vi "AddCurveArrDev.vi"(6 "ArrDevDat":T1[](array[typedef]), 8 "error in":errorcluster caption="entrée d'erreur (pas d'erreur)", 9 "CurPointInd":i32, 10 "Exper.lvclass In":refnum<class "Experiment.lvclass">, 11 "InterfaceIn":refnum<class "Interface.lvclass">) -> (0 "error out":errorcluster caption="sortie d'erreur", 3 "InterfaceOut":refnum<class "Interface.lvclass">)   [LabVIEW 2019, in "Interface.lvclass"]
uses:
  Interface.lvclass
  Experiment Class/Experiment.lvclass
  Experiment Class/ArrDevData.ctl
  CurveSetup.ctl
  AddCurveStatesArrDev.ctl
  ScanParams.ctl
  Interface.lvclass/Interface.ctl
panel:
  out "ReuseVarPar":bool
  out "DataFileName":path
  out "IndInGraphCrv":i32[](array[numeric])
  out "CurrDataQ":refnum<queue>[](array[refnum])
  out "CurrVarParQ":refnum<queue>[](array[refnum])
  out "Scan list":string[](array[string])
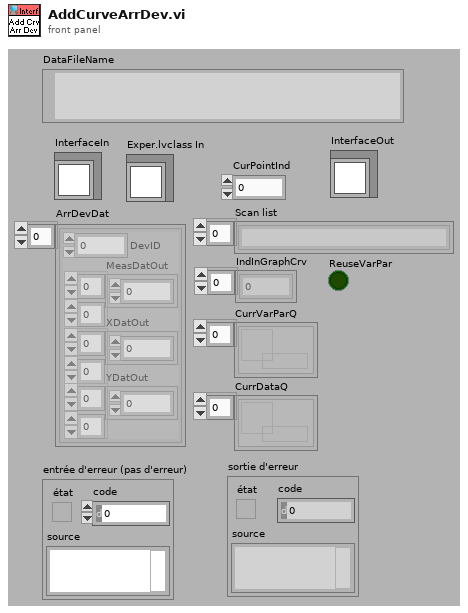
[diagram p1: front panel]
types:
  T1 = typedef "ArrDevData.ctl" = cluster{"MeasDatOut":dbl[][], "XDatOut":dbl[][], "YDatOut":dbl[][], "DevID":i32}
  T2 = typedef "Interface.lvclass/CurveSetup.ctl" = cluster{"CurveName":string, "YParam":string, "XParam":string, "ZParam ":string, "GroupName":string, "LinWdth":u8, "PntCol":u32, "LinCol":u32, "LablFor":u8, "XScale":u32, "YScale":u32, "Interpol":u8, "DisplayName":string, "FillType":i16, "LineStyle":u8, "PntStyle":u8, "BarTyp":u8, "GraphIndex":i32, "Visible":bool, "XScaleName":string, "YScaleName":string, "XYGraph_Ref":refnum<vi>, "Data Only":bool, "DataQ Ref":refnum<queue>, "XParQ Ref":refnum<queue>, "XParamInd":i32, "ScanInd":i32}
  T3 = typedef "Interface.lvclass/ScanParams.ctl" = cluster{"Entête":string, "Scan list":string[], "NbCourbe":i32, "IndCourbe":i64, "NomDon":string[], "Session ":i32, "Date":string, "Time":string, "VarParams":string[][], "UserName":string, "ScanTableSize":i32[], "VarPar list":string[], "DescKeyword":string}
  T4 = typedef "AddCurveStatesArrDev.ctl" = enum16{"CreateCurvePar", "AddToGraph", "AddToCrvParArr", "CreateDataQ", "UpdateGraph", "Error"}
  T5 = enum16{"open", "replace", "create", "open or create", "replace or create", "replace or create with confirmation"}
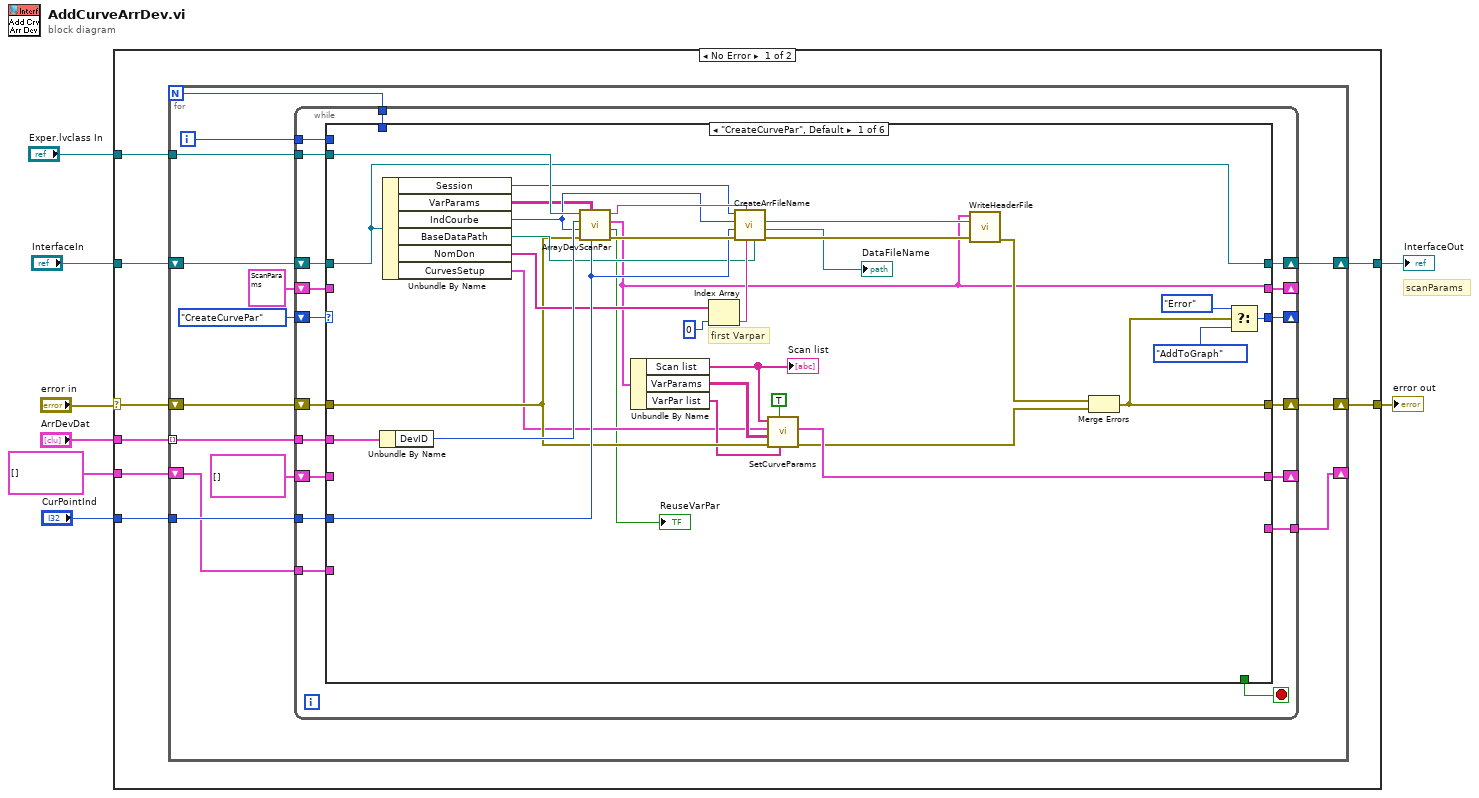
[diagram p0: block diagram]
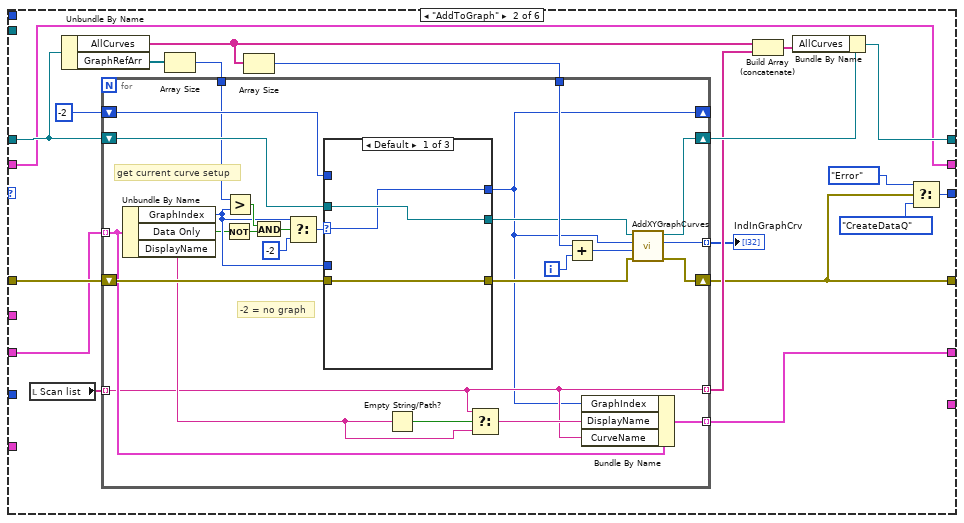
[diagram p2: hidden frame]
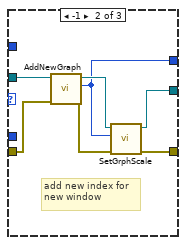
[diagram p3: hidden frame]
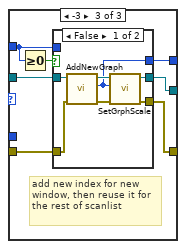
[diagram p4: hidden frame]
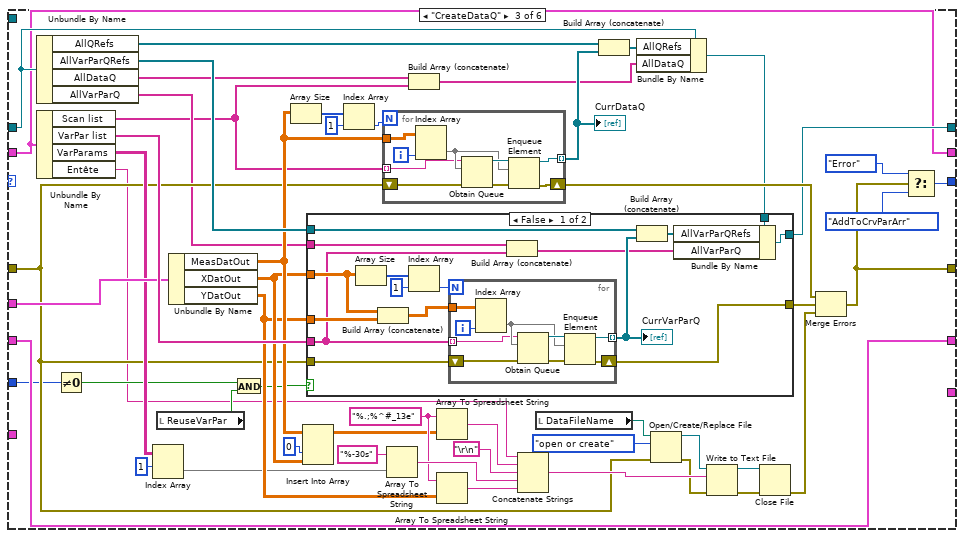
[diagram p6: hidden frame]
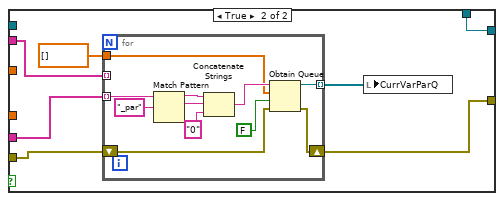
[diagram p7: hidden frame]
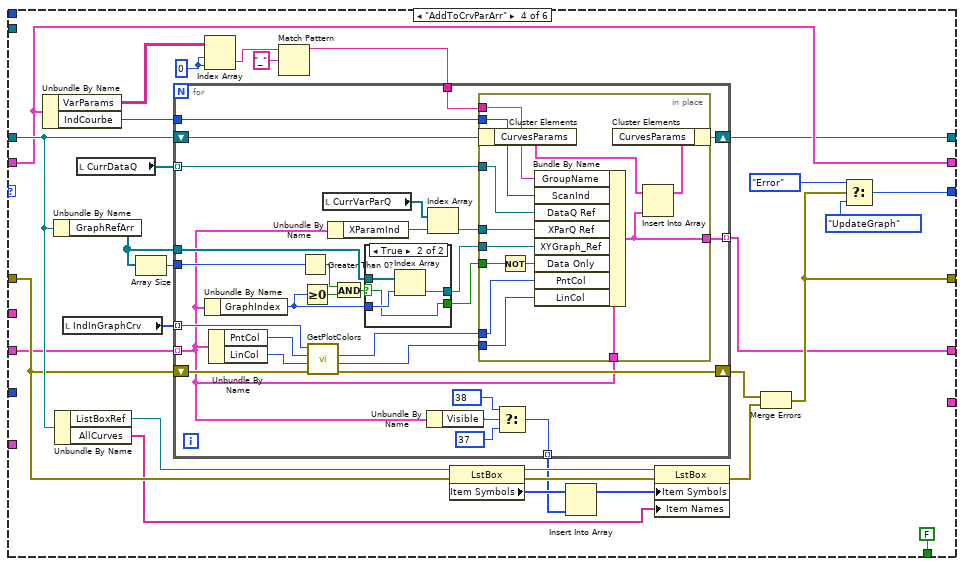
[diagram p8: hidden frame]
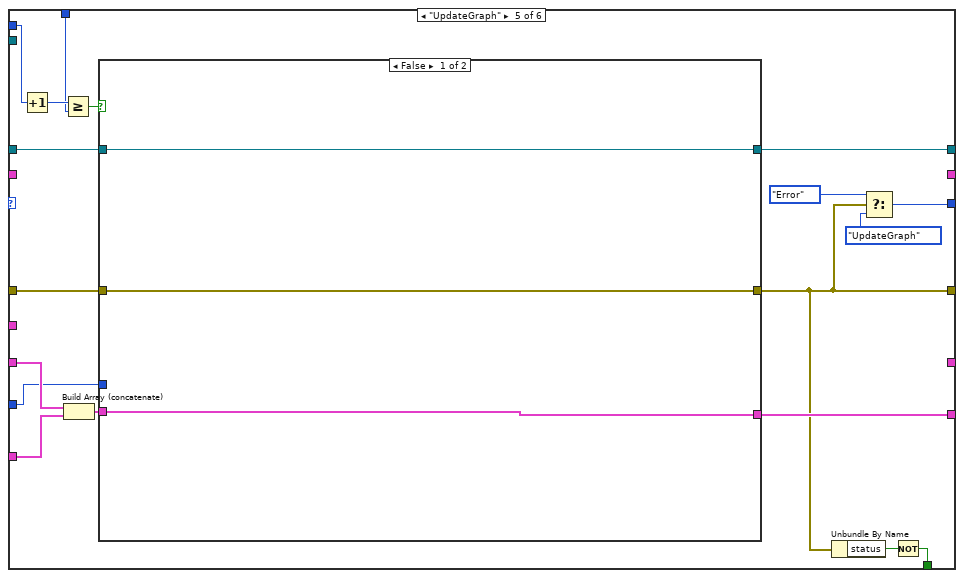
[diagram p10: hidden frame]
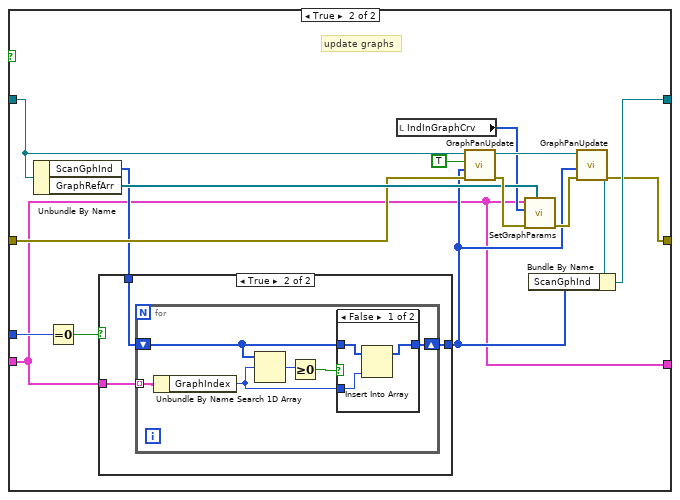
[diagram p11: hidden frame]
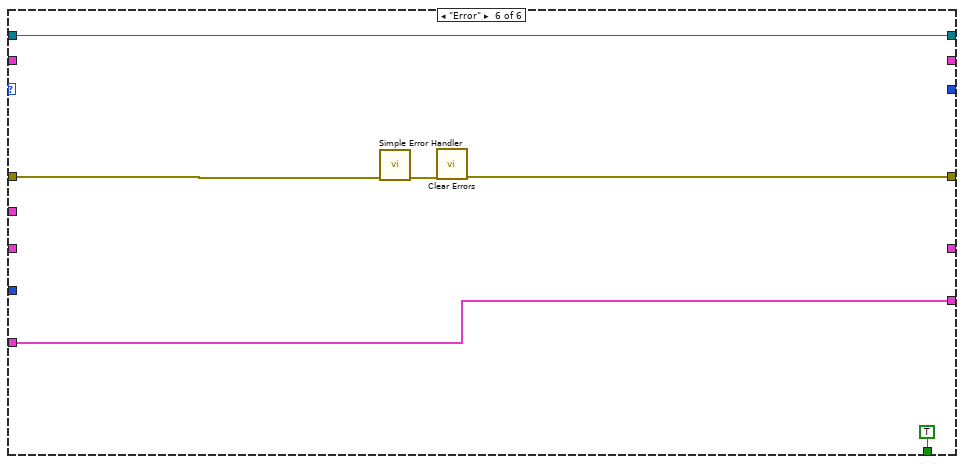
[diagram p14: hidden frame]
diagram:
  # "scanParams"
  n1 = case shown="No Error" "error in" {
    selector: "error in" -> [w16 w393]
    tunnel: [w15 w393] -> w7
    tunnel: "InterfaceIn" -> [w13 w392]
    tunnel: [w14 w392] -> w5
    tunnel: "ArrDevDat" -> [w12 _]
    tunnel: "Exper.lvclass In" -> [w11 _]
    tunnel: "CurPointInd" -> [w10 _]
    tunnel: T2[] [] ("CurveSetupsOut") -> [w9 _]
    frame No Error {
      n2 = for {
        N -> [w18]
        tunnel: w12 -> [w26] mode=indexing
        tunnel: w11 -> [w24]
        tunnel: w10 -> [w23]
        shift-right: [w29] -> w15
        shift-left: w16 -> [w30]
        shift-right: [w28] -> w14
        shift-left: w13 -> [w27]
        shift-right: [w19] -> _
        shift-left: w9 -> [w20]
        i -> [w17]
        n3 = while {
          shift-right: [w44] -> w29
          shift-left: w30 -> [w46]
          shift-right: [w45] -> _
          shift-left: AddCurveStatesArrDev."CreateCurvePar" ("Énum") -> [w47]
          shift-right: [w43] -> w28
          shift-left: w27 -> [w42]
          shift-right: [w41] -> _
          shift-left: T2[] [] ("CurveSetupsOut") -> [w40]
          tunnel: w26 -> [w39]
          tunnel: w24 -> [w38]
          tunnel: w23 -> [w37]
          shift-right: [w36] -> _
          shift-left: T3 {"Entête"="", "Scan list"=[], "NbCourbe"=1, "IndCourbe"=0, "NomDon"=["RTêta;", "X&Y;"], "Session "=0, "Date"="", "Time"="", "VarParams"=[], "UserName"="", "ScanTableSize"=[], "VarPar list"=[], "DescKeyword"=""} ("ScanPar") -> [w35]
          tunnel: w20 -> [w34]
          tunnel: [w33] -> w19
          tunnel: w18 -> [w32]
          tunnel: w17 -> [w31]
          stop <- w48 stop-if-true
          n4 = case shown="\"CreateCurvePar\", Default" w47 {
            tunnel: [_ _ _ FALSE w338 TRUE] -> w48
            tunnel: w46 -> [w64 w100 w168 w273 w352 w389]
            tunnel: w42 -> [w50 w96 w192 w285 w350 w387]
            tunnel: [w52 w84 w166 w264 w339 _] -> w45
            tunnel: [w54 w82 w164 w261 w337 w388] -> w44
            tunnel: [w50 w98 w194 w260 w351 w387] -> w43
            tunnel: [w60 w87 w169 w259 _ _] -> w41
            tunnel: w40 -> [_ w94 w169 w267 w349 _]
            tunnel: w39 -> [w79 _ w198 _ _ _]
            tunnel: w38 -> [w80 _ _ _ _ _]
            tunnel: w37 -> [w73 _ w162 _ w335 _]
            tunnel: [w63 w81 w163 w268 _ _] -> w36
            tunnel: w35 -> [_ w81 w163 w268 _ _]
            tunnel: w34 -> [_ _ _ _ w348 w386]
            tunnel: [_ _ _ _ w347 w386] -> w33
            tunnel: w32 -> [_ _ _ _ w344 _]
            tunnel: w31 -> [_ _ _ _ w343 _]
            frame "CreateCurvePar", Default {
              # "first Varpar"
              n5 = Unbundle By Name(w79) -> ("DevID"=w78:i32)
              n6 = Unbundle By Name(w50) -> ("Session"=w69:i32, "VarParams"=w66:string[][], "IndCourbe"=w72:i64, "BaseDataPath"=w68:path, "NomDon"=w65:string[], "CurvesSetup"=w57:T2[])
              n7 = call "ArrayDevScanPar.vi"("CurPointInd"=w73, "VarParams"=w66, "error in"=w64, "IndCourbe"=w72, "DevID"=w78, "Experiment.lvclass In"=w80) -> ("error out"=w77:errorcluster, "ReuseVarPar"=→"ReuseVarPar":bool, "ScanPar"=w63:T3, "FileNmDTString"=w76:string)  [unwired: 2 in]
              n8 = Unbundle By Name(w63) -> ("Scan list"=w58:string[], "VarParams"=w62:string[][], "VarPar list"=w61:string[])
              "Scan list" <- w58
              n9 = Index Array(array=w65, index=0 ("indice (ligne)")) -> (element=w74:string)
              n10 = call "CreateArrFileName.vi"("BaseDataPath"=w68, "VarParName"=w74, "Date"=w76, "error in (no error)"=w77, "PointIndex"=w73, "ScanIndex"=w72, "SessionInd"=w69) -> ("error out"=w71:errorcluster, "DataFileName"=→"DataFileName":path, "HeadersFileName"=w70:path)  [unwired: 2 in]
              n11 = call "SetCurveParams.vi"("VarPar list"=w61, "AllowDef"=TRUE, "error in (no error)"=w64, "VarParams"=w62, "CurveSetupsIn"=w57, "CurveNames"=w58) -> ("error out"=w59:errorcluster, "CurveSetupsOut"=w60:T2[])  [unwired: 4 in]
              n12 = call "WriteHeaderFile.vi"("error in (no error)"=w71, "HeadersFileName"=w70, "ScanPar"=w63) -> ("error out"=w67:errorcluster)  [unwired: 8 in]
              n13 = Merge Errors(w67, w59) -> (w54:errorcluster)
              n14 = Select(t=AddCurveStatesArrDev."Error" ("Énum"), s=w54, f=AddCurveStatesArrDev."AddToGraph" ("Énum")) -> (s? t:f=w52:T4)
            }
            frame "AddToGraph" {
              n15 = local read "Scan list"() -> (w88:string[])
              n16 = Unbundle By Name(w96) -> ("AllCurves"=w91:string[], "GraphRefArr"=w93:refnum<vi>[])
              n17 = Array Size(array=w93) -> (size(s)=w92:i32)
              n18 = Array Size(array=w91) -> (size(s)=w95:i32)
              n19 = for {
                tunnel: w94 -> [w118] mode=indexing
                shift-right: [w102] -> _
                shift-left: -2 ("NewGraphInd") -> [w117]
                shift-right: [w106] -> w99
                shift-left: w96 -> [w116]
                tunnel: w95 -> [w108]
                tunnel: w92 -> [w115]
                tunnel: [w110] -> w89 mode=indexing
                tunnel: [w114] -> w87 mode=indexing
                tunnel: w88 -> [w110] mode=indexing
                shift-right: [w104] -> w82
                shift-left: w100 -> [w119]
                tunnel: [w101] -> w86 mode=indexing
                i -> [w109]
                # "-2 = no graph"
                # "get current curve setup"
                n20 = Unbundle By Name(w118) -> ("GraphIndex"=w125:i32, "Data Only"=w122:bool, "DisplayName"=w112:string)
                n21 = Not(x=w122) -> (.not. x?=w121:bool)
                n22 = Greater?(x=w115, y=w125) -> (0:w126:bool)
                n23 = And(x=w126, y=w121) -> (x .and. y?=w120:bool)
                n24 = Select(t=w125, s=w120, f=-2 ("cas faux")) -> (s? t:f=w123:i32)
                n25 = case shown="Default" w123 {
                  selector: w123 -> [w127 _ _]
                  tunnel: w125 -> [_ _ _]
                  tunnel: [w127 w130 w139] -> w102
                  tunnel: w116 -> [w129 w136 w143]
                  tunnel: w119 -> [w128 w135 w142]
                  tunnel: [w129 w133 w141] -> w107
                  tunnel: [w128 w131 w140] -> w105
                  tunnel: w117 -> [_ _ w137]
                  frame Default {
                  }
                  frame -1 {
                    # "add new index for new window"
                    n26 = call "AddNewGraph.vi"("error in (no error)"=w135, "Interface en entrée"=w136) -> ("error out"=w132:errorcluster, "NewGraphInd"=w130:i32, "Interface en sortie"=w134:refnum<class "Interface.lvclass">)  [unwired: 7 in]
                    n27 = call "SetGrphScale.vi"("error in (no error)"=w132, "GraphIndex"=w130, "Interface en entrée"=w134) -> ("error out"=w131:errorcluster, "Interface en sortie"=w133:refnum<class "Interface.lvclass">)  [unwired: 7 in]
                  }
                  frame -3 {
                    # "add new index for new window, then reuse it for the rest of scanlist"
                    n28 = Greater Or Equal To 0?(x=w137) -> (x >= 0?=w138:bool)
                    n29 = case shown="False" w138 {
                      tunnel: w143 -> [w150 w153]
                      tunnel: w142 -> [w149 w152]
                      tunnel: [w147 w153] -> w141
                      tunnel: [w145 w152] -> w140
                      tunnel: [w144 w151] -> w139
                      tunnel: w137 -> [_ w151]
                      frame False {
                        n30 = call "AddNewGraph.vi"("error in (no error)"=w149, "Interface en entrée"=w150) -> ("error out"=w146:errorcluster, "NewGraphInd"=w144:i32, "Interface en sortie"=w148:refnum<class "Interface.lvclass">)  [unwired: 7 in]
                        n31 = call "SetGrphScale.vi"("error in (no error)"=w146, "GraphIndex"=w144, "Interface en entrée"=w148) -> ("error out"=w145:errorcluster, "Interface en sortie"=w147:refnum<class "Interface.lvclass">)  [unwired: 7 in]
                      }
                      frame True {
                      }
                    }
                  }
                }
                n32 = Empty String/Path?(string/path=w112) -> (empty?=w113:bool)
                n33 = Select(t=w110, s=w113, f=w112) -> (s? t:f=w111:string)
                n34 = Add(x=w108, y=w109) -> (x+y=w103:i32)
                n35 = Bundle By Name(cluster=w118, "GraphIndex"=w102, "DisplayName"=w111, "CurveName"=w110) -> (w114:T2)
                n36 = call "AddXYGraphCurves.vi"("error in (no error)"=w105, "CurvIndex"=w103, "GraphIndex"=w102, "Interface en entrée"=w107) -> ("error out"=w104:errorcluster, "IndInGrphCrv"=w101:i32, "Interface en sortie"=w106:refnum<class "Interface.lvclass">)  [unwired: 5 in]
              }
              "IndInGraphCrv" <- w86
              n37 = Build Array (concatenate)(w91, w89) -> (w90:string[])
              n38 = Bundle By Name(cluster=w99, "AllCurves"=w90) -> (w98:refnum<class "Interface.lvclass">)
              n39 = Select(t=AddCurveStatesArrDev."Error" ("Énum"), s=w82, f=AddCurveStatesArrDev."CreateDataQ" ("Énum")) -> (s? t:f=w84:T4)
            }
            frame "CreateDataQ" {
              w185 = "%.;%^#_13e" ("chaîne de format")
              n40 = Unbundle By Name(w192) -> ("AllQRefs"=w193:refnum<queue>[], "AllVarParQRefs"=w200:refnum<queue>[], "AllDataQ"=w156:string[], "AllVarParQ"=w158:string[])
              n41 = Unbundle By Name(w163) -> ("Scan list"=w155:string[], "VarPar list"=w199:string[], "VarParams"=w177:string[][], "Entête"=w157:string)
              n42 = Not Equal To 0?(x=w162) -> (x != 0?=w159:bool)
              n43 = Index Array(array=w177, index (row)=1 ("indice (ligne)")) -> (element=w175:string[])  [unwired: 1 in]
              n44 = local read "ReuseVarPar"() -> (w160:bool)
              n45 = Unbundle By Name(w198) -> ("MeasDatOut"=w190:dbl[][], "XDatOut"=w180:dbl[][], "YDatOut"=w178:dbl[][])
              n46 = And(x=w159, y=w160) -> (x .and. y?=w161:bool)
              n47 = Array Size(array=w190) -> (size(s)=w205:i32[])
              n48 = Insert Into Array(array=w190, index (col)=0 ("indice désactivé (col)"), new element=w180) -> (w179:dbl[][])  [unwired: 1 in]
              n49 = Index Array(array=w205, index=1 ("indice")) -> (element=w203:i32)
              n50 = for {
                N: w203 -> [_]
                tunnel: w190 -> [w256]
                shift-right: [w257] -> w196
                shift-left: w168 -> [w251]
                tunnel: [w252] -> w202 mode=indexing
                tunnel: w155 -> [w250] mode=indexing
                i -> [w249]
                n51 = Index Array(array=w256, index (col)=w249) -> (element=w253:dbl[])  [unwired: 1 in]
                n52 = Obtain Queue(name (unnamed)=w250, element data type=w253, error in (no error)=w251) -> (queue out=w255:refnum<queue>, error out=w254:errorcluster)  [unwired: 2 in, 1 out]
                n53 = Enqueue Element(queue=w255, element=w253, error in (no error)=w254) -> (queue out=w252:refnum<queue>, error out=w257:errorcluster)  [unwired: 1 in, 1 out]
              }
              "CurrDataQ" <- w202
              n54 = Array To Spreadsheet String(array=w175, 3:"%-30s" ("chaîne de format")) -> (spreadsheet string=w188:string)  [unwired: 1 in]
              n55 = Build Array (concatenate)(w156, w155) -> (w154:string[])
              n56 = Array To Spreadsheet String(array=w179, 3:w185) -> (spreadsheet string=w186:string)  [unwired: 1 in]
              n57 = Array To Spreadsheet String(array=w178, 3:w185) -> (spreadsheet string=w181:string)  [unwired: 1 in]
              n58 = Concatenate Strings(w157, w186, "\r\n", w188, w181) -> (w182:string)
              n59 = local read "DataFileName"() -> (w171:path)
              n60 = Build Array (concatenate)(w193, w202) -> (w201:refnum<queue>[])
              n61 = Bundle By Name(cluster=w192, "AllQRefs"=w201, "AllDataQ"=w154) -> (w195:refnum<class "Interface.lvclass">)
              n62 = case shown="False" w161 {
                tunnel: w180 -> [w211 _]
                tunnel: w200 -> [w210 _]
                tunnel: w178 -> [w216 _]
                tunnel: w199 -> [w208 w236]
                tunnel: w168 -> [w215 w234]
                tunnel: [w209 w231] -> w197
                tunnel: w195 -> [w214 w237]
                tunnel: [w213 w237] -> w194
                tunnel: w158 -> [w207 w235]
                frame False {
                  n63 = Array Size(array=w211) -> (size(s)=w219:i32[])
                  n64 = Build Array (concatenate)(w211, w216) -> (w217:dbl[][])
                  n65 = Index Array(array=w219, index=1 ("indice")) -> (element=w221:i32)
                  n66 = for {
                    N: w221 -> [_]
                    tunnel: w217 -> [w229]
                    shift-right: [w230] -> w209
                    shift-left: w215 -> [w224]
                    tunnel: [w225] -> w218 mode=indexing
                    tunnel: w208 -> [w223] mode=indexing
                    i -> [w222]
                    n67 = Index Array(array=w229, index (col)=w222) -> (element=w226:dbl[])  [unwired: 1 in]
                    n68 = Obtain Queue(name (unnamed)=w223, element data type=w226, error in (no error)=w224) -> (queue out=w228:refnum<queue>, error out=w227:errorcluster)  [unwired: 2 in, 1 out]
                    n69 = Enqueue Element(queue=w228, element=w226, error in (no error)=w227) -> (queue out=w225:refnum<queue>, error out=w230:errorcluster)  [unwired: 1 in, 1 out]
                  }
                  "CurrVarParQ" <- w218
                  n70 = Build Array (concatenate)(w207, w208) -> (w206:string[])
                  n71 = Build Array (concatenate)(w210, w218) -> (w212:refnum<queue>[])
                  n72 = Bundle By Name(cluster=w214, "AllVarParQRefs"=w212, "AllVarParQ"=w206) -> (w213:refnum<class "Interface.lvclass">)
                }
                frame True {
                  n73 = for {
                    tunnel: w236 -> [w247] mode=indexing
                    tunnel: w235 -> [_] mode=indexing
                    tunnel: [w242] -> w232 mode=indexing
                    shift-right: [w240] -> w231
                    shift-left: w234 -> [w241]
                    tunnel: dbl[] [] ("sous-tableau") -> [w239]
                    n74 = Match Pattern(string=w247, regular expression="_par" ("expression régulière")) -> (before substring=w246:string, match substring=w245:string)  [unwired: 1 in, 2 out]
                    n75 = Concatenate Strings(w246, w245, "0" ("chaîne")) -> (w243:string)
                    n76 = Obtain Queue(name (unnamed)=w243, element data type=w239, create if not found? (T)=FALSE ("créer si introuvable ? (V)"), error in (no error)=w241) -> (queue out=w242:refnum<queue>, error out=w240:errorcluster)  [unwired: 1 in, 1 out]
                  }
                  n77 = local write "CurrVarParQ"(w232) -> ()
                }
              }
              n78 = Open/Create/Replace File(file path (use dialog)=w171, error in=w168, operation (0:open)=T5."open or create" ("opération (0 : open)")) -> (refnum out=w170:refnum<file>, error out=w172:errorcluster)  [unwired: 3 in, 1 out]
              n79 = Write to Text File(file (use dialog)=w170, text=w182, error in=w172) -> (refnum out=w184:refnum<file>, error out=w183:errorcluster)  [unwired: 1 in, 1 out]
              n80 = Close File(refnum=w184, error in=w183) -> (error out=w174:errorcluster)  [unwired: 1 out]
              n81 = Merge Errors(w196, w197, w174) -> (w164:errorcluster)
              n82 = Select(t=AddCurveStatesArrDev."Error" ("Énum"), s=w164, f=AddCurveStatesArrDev."AddToCrvParArr" ("Énum")) -> (s? t:f=w166:T4)
            }
            frame "AddToCrvParArr" {
              w280 = 0 ("indice désactivé (col)")
              n83 = Unbundle By Name(w268) -> ("VarParams"=w281:string[][], "IndCourbe"=w282:i64)
              n84 = Unbundle By Name(w285) -> ("GraphRefArr"=w284:refnum<vi>[])
              n85 = Unbundle By Name(w285) -> ("ListBoxRef"=w276:refnum<vi>, "AllCurves"=w265:string[])
              n86 = local read "IndInGraphCrv"() -> (w287:i32[])
              n87 = local read "CurrDataQ"() -> (w283:refnum<queue>[])
              n88 = Array Size(array=w284) -> (size(s)=w286:i32)
              n89 = Index Array(array=w281, index (row)=w280, index (col)=w280) -> (element=w279:string)
              n90 = Match Pattern(string=w279, regular expression="_" ("expression régulière")) -> (before substring=w277:string)  [unwired: 1 in, 3 out]
              n91 = for {
                tunnel: w267 -> [w291] mode=indexing
                tunnel: w287 -> [w308] mode=indexing
                tunnel: w284 -> [w305]
                tunnel: w286 -> [w304]
                tunnel: w283 -> [w302] mode=indexing
                tunnel: w282 -> [w297]
                tunnel: w277 -> [w290]
                tunnel: [w293] -> w271 mode=indexing
                shift-right: [w292] -> w266
                shift-left: w273 -> [w313]
                shift-right: [w289] -> w260
                shift-left: w285 -> [w316]
                tunnel: [w288] -> w259 mode=indexing
                n92 = Unbundle By Name(w291) -> ("GraphIndex"=w312:i32)
                n93 = Unbundle By Name(w291) -> ("PntCol"=w314:u32, "LinCol"=w315:u32)
                n94 = Greater Than 0?(x=w304) -> (x > 0?=w309:bool)
                n95 = Greater Or Equal To 0?(x=w312) -> (x >= 0?=w310:bool)
                n96 = call "GetPlotColors.vi"("ErrorIn(No Error)"=w313, "Color2In"=w315, "Color1In"=w314, "ColorIndex"=w308) -> ("sortie d'erreur"=w292:errorcluster, "Color2Out"=w307:u32, "Color1Out"=w306:u32)  [unwired: 4 in, 1 out]
                n97 = local read "CurrVarParQ"() -> (w300:refnum<queue>[])
                n98 = Unbundle By Name(w291) -> ("XParamInd"=w301:i32)
                n99 = And(x=w309, y=w310) -> (x .and. y?=w311:bool)
                n100 = case shown="True" w311 {
                  selector: w311 -> [w317 w318]
                  tunnel: [_ w321] -> w298
                  tunnel: w305 -> [_ w320]
                  tunnel: w312 -> [_ w319]
                  tunnel: [w317 w318] -> w303
                  frame False {
                  }
                  frame True {
                    n101 = Index Array(array=w320, index=w319) -> (element=w321:refnum<vi>)
                  }
                }
                n102 = Unbundle By Name(w291) -> ("Visible"=w296:bool)
                n103 = Index Array(array=w300, index=w301) -> (element=w299:refnum<queue>)
                n104 = in-place {
                  in-place-border: w307 -> [w325]
                  in-place-border: w306 -> [w324]
                  in-place-border: w298 -> [w332]
                  in-place-border: w303 -> [w331]
                  in-place-border: w302 -> [w330]
                  in-place-border: w299 -> [w329]
                  in-place-border: w297 -> [w327]
                  in-place-border: w291 -> [w328]
                  in-place-border: w290 -> [w326]
                  in-place-border: [w322] -> w288
                  n105 = in-place-cluster #1(w316) -> ("CurvesParams"=w334:T2[])
                  n106 = Not(x=w331) -> (.not. x?=w323:bool)
                  n107 = Bundle By Name(cluster=w328, "GroupName"=w326, "ScanInd"=w327, "DataQ Ref"=w330, "XParQ Ref"=w329, "XYGraph_Ref"=w332, "Data Only"=w323, "PntCol"=w324, "LinCol"=w325) -> (w322:T2)
                  n108 = Insert Into Array(array=w334, new element=w322) -> (w333:T2[])  [unwired: 1 in]
                  n109 = in-place-cluster #1("CurvesParams"=w333) -> (w289:refnum<class "Interface.lvclass">)
                }
                n110 = Select(t=38, s=w296, f=37) -> (s? t:f=w293:i32)
              }
              n111 = property on="Nœud de propriété" class="LstBox"(reference=w276, error in=w273) -> (reference out=w275:refnum<vi>, error out=w274:errorcluster, "Item Symbols"=w272:i32[])
              n112 = Insert Into Array(array=w272, new element=w271) -> (w270:i32[])  [unwired: 1 in]
              n113 = property on="Nœud de propriété" class="LstBox"(reference=w275, error in=w274, "Item Symbols"=w270, "Item Names"=w265) -> (error out=w269:errorcluster)  [unwired: 1 out]
              n114 = Merge Errors(w266, w269) -> (w261:errorcluster)
              n115 = Select(t=AddCurveStatesArrDev."Error" ("Énum"), s=w261, f=AddCurveStatesArrDev."UpdateGraph" ("Énum")) -> (s? t:f=w264:T4)
            }
            frame "UpdateGraph" {
              n116 = Increment(x=w343) -> (x+1=w345:i32)
              n117 = Greater Or Equal?(x=w345, y=w344) -> (x >= y?=w342:bool)
              n118 = Build Array (concatenate)(w349, w348) -> (w346:T2[])
              n119 = case shown="False" w342 {
                tunnel: [w353 w361] -> w337
                tunnel: w352 -> [w353 w367]
                tunnel: [w354 w364] -> w351
                tunnel: w350 -> [w354 w370]
                tunnel: [w355 w356] -> w347
                tunnel: w346 -> [w355 w356]
                tunnel: w335 -> [_ w358]
                frame False {
                }
                frame True {
                  # "update graphs"
                  n120 = Unbundle By Name(w370) -> ("ScanGphInd"=w360:i32[], "GraphRefArr"=w368:refnum<vi>[])
                  n121 = Equal To 0?(x=w358) -> (x = 0?=w357:bool)
                  n122 = case shown="True" w357 {
                    tunnel: w356 -> [_ w375]
                    tunnel: w360 -> [w372 w374]
                    tunnel: [w372 w373] -> w359
                    frame False {
                    }
                    frame True {
                      n123 = for {
                        shift-right: [w379] -> w373
                        shift-left: w374 -> [w380]
                        tunnel: w375 -> [w377] mode=indexing
                        n124 = Unbundle By Name(w377) -> ("GraphIndex"=w376:i32)
                        n125 = Search 1D Array(1D array=w380, element=w376) -> (index of element=w381:i32)  [unwired: 1 in]
                        n126 = Greater Or Equal To 0?(x=w381) -> (x >= 0?=w378:bool)
                        n127 = case shown="False" w378 {
                          tunnel: w380 -> [w384 w385]
                          tunnel: [w383 w385] -> w379
                          tunnel: w376 -> [w382 _]
                          frame False {
                            n128 = Insert Into Array(array=w384, new element=w382) -> (w383:i32[])  [unwired: 1 in]
                          }
                          frame True {
                          }
                        }
                      }
                    }
                  }
                  n129 = local read "IndInGraphCrv"() -> (w362:i32[])
                  n130 = call "GraphPanUpdate.vi"("error in (no error)"=w367, "GraphInd"=w359, "DeferUpdate"=TRUE, "Interface en entrée"=w370) -> ("error out"=w369:errorcluster, "Interface en sortie"=w366:refnum<class "Interface.lvclass">)  [unwired: 6 in]
                  n131 = call "SetGraphParams.vi"("GraphRefArr"=w368, "error in"=w369, "CuurGrphCrvInd"=w362, "CurveSetupsIn"=w356) -> ("error out"=w365:errorcluster)  [unwired: 7 in]
                  n132 = call "GraphPanUpdate.vi"("error in (no error)"=w365, "GraphInd"=w359, "Interface en entrée"=w366) -> ("error out"=w361:errorcluster, "Interface en sortie"=w363:refnum<class "Interface.lvclass">)  [unwired: 7 in]
                  n133 = Bundle By Name(cluster=w363, "ScanGphInd"=w359) -> (w364:refnum<class "Interface.lvclass">)
                }
              }
              n134 = Unbundle By Name(w337) -> ("status"=w336:bool)
              n135 = Select(t=AddCurveStatesArrDev."Error" ("Énum"), s=w337, f=AddCurveStatesArrDev."UpdateGraph" ("Énum")) -> (s? t:f=w339:T4)
              n136 = Not(x=w336) -> (.not. x?=w338:bool)
            }
            frame "Error" {
              n137 = call <vilib>:"Simple Error Handler.vi"("error in (no error)"=w389) -> ("error out"=w390:errorcluster)  [unwired: 4 in, 4 out]
              n138 = call <vilib>:"Clear Errors.vi"("error in (no error)"=w390) -> ("error out"=w388:errorcluster)  [unwired: 5 in, 1 out]
            }
          }
        }
      }
    }
    frame Error {
    }
  }
  "error out" <- w7
  "InterfaceOut" <- w5
